vi "Generate Trajectory.vi"   [LabVIEW 2023]
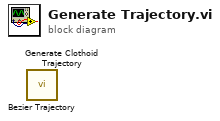
[diagram p0: block diagram]
diagram:
  n1 = call "Bezier Trajectory.vi"() -> ()  [unwired: 8 in, 4 out]
  n2 = call "Generate Clothoid Trajectory.vi"() -> ()  [unwired: 8 in, 4 out]
